vi "LoggingSystem.vi"(0 "Array":string[][](array[string]), 1 "Path":path) -> ()   [LabVIEW 2020]
uses:
  <vilib>/Utility/NIReport.llb/Report Type.ctl
  <vilib>/Utility/NIReport.llb/Append Text Table to Report (wrap).vi
  <vilib>/Utility/NIReport.llb/NI_report.lvclass
  <vilib>/Utility/NIReport.llb/Excel/NI_Excel.lvclass
  <vilib>/Utility/NIReport.llb/NI_ReportGenerationCore.lvlib
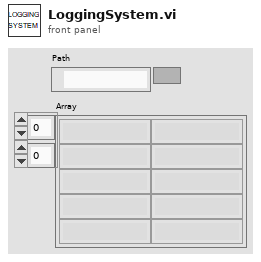
[diagram p1: front panel]
types:
  T1 = typedef "NI_ReportGenerationCore.lvlib/Report Type.ctl" = enum16{"HTML", "Word", "Excel"}
  T2 = enum16{"maximized", "minimized", "normal", "no change"}
  T3 = cluster{"position (excel)":cluster{"row":i32, "column":i32}, "name (excel)":string, "bookmark (word)":string}
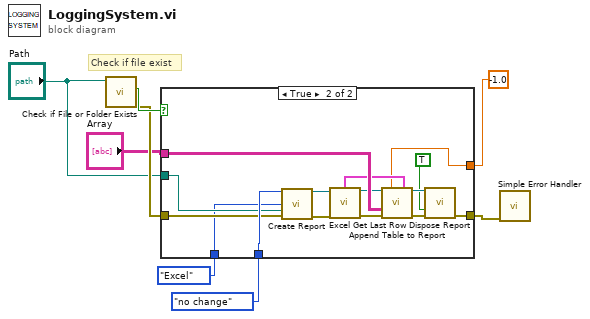
[diagram p0: block diagram]
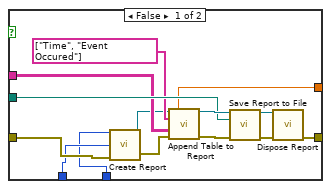
[diagram p2: hidden frame]
diagram:
  # "Check if file exist"
  n1 = call <vilib>:"Check if File or Folder Exists.vi"("path"="Path") -> ("error out"=w7:errorcluster, "file or folder exists?"=w8:bool)  [unwired: 8 in, 1 out]
  n2 = case shown="True" w8 {
    tunnel: w7 -> [w12 w26]
    tunnel: "Path" -> [w17 w27]
    tunnel: "Array" -> [w15 w33]
    tunnel: [w18 w34] -> w6
    tunnel: -1.0 ("column width (1)") -> [w14 w29]
    tunnel: T2."no change" ("window state (normal)") -> [w10 w28]
    tunnel: Report_Type."Excel" ("report type") -> [w11 w25]
    frame False {
      n3 = call <vilib>:"Create Report.vi"("window state (normal)"=w10, "report type"=w11, "error in (no error)"=w12) -> ("report out"=w9:refnum<class "NI_report.lvclass">, "error out"=w13:errorcluster)  [unwired: 11 in]
      n4 = call-poly <vilib>:"Append Table to Report.vi"("report in"=w9, "column width (1)"=w14, "column headers"=string[] ["Time", "Event Occured"], "text data"=w15, "error in (no error)"=w13) -> ("report out"=w21:refnum<class "NI_report.lvclass">, "error out"=w22:errorcluster)  [unwired: 4 in, 5 out]
      n5 = call-dynamic "Save Report to File.vi"("report in"=w21, "report file path"=w17, "error in (no error)"=w22) -> ("report out"=w20:refnum<class "NI_report.lvclass">, "error out"=w19:errorcluster)  [unwired: 2 in, 9 out]
      n6 = call-dynamic "Dispose Report.vi"("report in"=w20, "error in (no error)"=w19) -> ("error out"=w18:errorcluster)  [unwired: 3 in, 10 out]
    }
    frame True {
      n7 = call <vilib>:"Create Report.vi"("window state (normal)"=w28, "report type"=w25, "template (empty)"=w27, "error in (no error)"=w26) -> ("report out"=w24:refnum<class "NI_report.lvclass">, "error out"=w23:errorcluster)  [unwired: 10 in]
      n8 = call <vilib>:"Excel Get Last Row.vi"("report in"=w24, "error in (no error)"=w23) -> ("report out"=w32:refnum<class "NI_report.lvclass">, "MS Office parameters out"=w30:T3, "error out"=w31:errorcluster)  [unwired: 1 in, 10 out]
      n9 = call-poly <vilib>:"Append Table to Report.vi"("report in"=w32, "column width (1)"=w29, "MS Office parameters"=w30, "text data"=w33, "error in (no error)"=w31) -> ("report out"=w36:refnum<class "NI_report.lvclass">, "error out"=w37:errorcluster)  [unwired: 4 in, 5 out]
      n10 = call-dynamic "Dispose Report.vi"("report in"=w36, "save changes? (F)"=TRUE, "error in (no error)"=w37) -> ("error out"=w34:errorcluster)  [unwired: 2 in, 10 out]
    }
  }
  n11 = call <vilib>:"Simple Error Handler.vi"("error in (no error)"=w6) -> ()  [unwired: 1 in, 8 out]
